vi "api_mqttPublish.vi"(0 "mqtt.lvclass in":refnum<class "mqtt.lvclass">, 5 "topic":string, 7 "value":string, 9 "QoS (At most once)":T3, 11 "error in (no error)":errorcluster, 12 "retain(F)":bool, 13 "duplicate(F)":bool, 14 "messageID":u16) -> (4 "mqtt.lvclass out":refnum<class "mqtt.lvclass">, 6 "success":bool, 15 "error out":errorcluster)   [LabVIEW 2018, in "labview-mqtt.lvlib" / "mqtt.lvclass"]
uses:
  mqtt.lvclass
  mqttTypedef/mqttQOSlevel.ctl
  mqttTypedef/mqttRXdataCluster.ctl
  mqttTypedef/mqttFixedHeaderResponse.ctl
  mqttTypedef/mqttMessageType.ctl
  mqttCmd/mqttCmdPublish/mqttCmdPublish.lvclass
  D:/OneDrive/_WorkingOn/IECube/MQTT LabVIEW/mqtt-LabVIEW-master-yao/src/class/mqtt/mqttCmd/mqttCmd.lvclass
  mqttCmd/mqttCmdPublish/mqttCmdPublish.lvclass/mqttCmdPublish.ctl
  mqttCmd/mqttCmd.lvclass/mqttCmd.ctl
  mqttCmd/mqttCmd.lvclass
  labview-mqtt.lvlib
panel:
  out "notification":T1
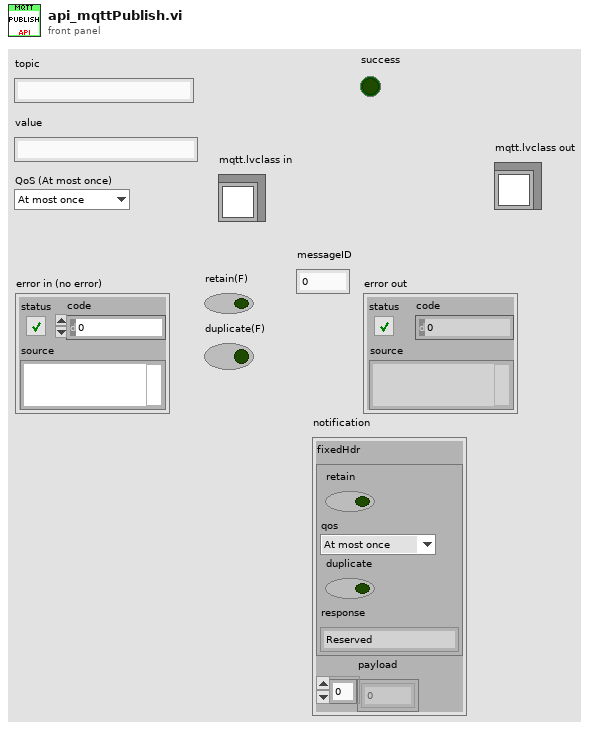
[diagram p1: front panel]
types:
  T1 = typedef "labview-mqtt.lvlib/mqttRXdataCluster.ctl" = cluster{"fixedHdr":T2, "payload":u8[]}
  T2 = typedef "labview-mqtt.lvlib/mqttFixedHeaderResponse.ctl" = cluster{"retain":bool, "qos":T3, "duplicate":bool, "response":T4}
  T3 = typedef "labview-mqtt.lvlib/mqttQOSlevel.ctl" = enum8{"At most once", "At least once", "Exactly once", "Reserved"}
  T4 = typedef "labview-mqtt.lvlib/mqttMessageType.ctl" = enum32{"Reserved", "CONNECT", "CONNACK", "PUBLISH", "PUBACK", "PUBREC", "PUBREL", "PUBCOMP", "SUBSCRIBE", "SUBACK", "UNSUBSCRIBE", "UNSUBACK", "PINGREQ", "PINGRESP", "DISCONNECT", "Reserved2"}
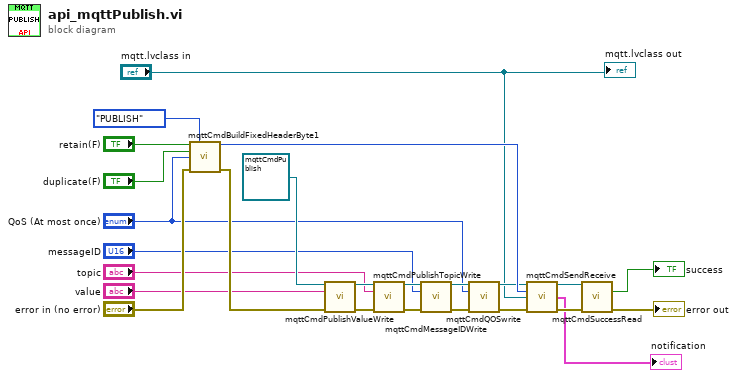
[diagram p0: block diagram]
diagram:
  n1 = call "mqttCmdBuildFixedHeaderByte1.vi"("retain(F)"="retain(F)", "MessageType"=mqttMessageType."PUBLISH", "duplicate(F)"="duplicate(F)", "QoS (At most once)"="QoS (At most once)", "error in (no error)"="error in (no error)") -> ("byte1"=w24:u8, "error out"=w20:errorcluster)  [unwired: 9 in]
  n2 = call "mqttCmdPublishValueWrite.vi"("mqttPublish in"=refnum<class "mqttCmdPublish.lvclass"> refnum ("mqttPublish.lvclass"), "value"="value", "error in (no error)"=w20) -> ("mqttPublish out"=w17:refnum<class "mqttCmdPublish.lvclass">, "error out"=w19:errorcluster)  [unwired: 11 in]
  n3 = call "mqttCmdPublishTopicWrite.vi"("mqttPublish in"=w17, "topic"="topic", "error in (no error)"=w19) -> ("mqttPublish out"=w11:refnum<class "mqttCmdPublish.lvclass">, "error out"=w12:errorcluster)  [unwired: 11 in]
  n4 = call "mqttCmdMessageIDWrite.vi"("mqttBrokerCommand in"=w11, "messageID"="messageID", "error in (no error)"=w12) -> ("mqttBrokerCommand out"=w7:refnum<class "mqttCmdPublish.lvclass">, "error out"=w9:errorcluster)  [unwired: 11 in]
  n5 = call "mqttCmdQOSwrite.vi"("mqttBrokerCommand in"=w7, "QoS"="QoS (At most once)", "error in (no error)"=w9) -> ("mqttBrokerCommand out"=w6:refnum<class "mqttCmdPublish.lvclass">, "error out"=w8:errorcluster)  [unwired: 11 in]
  n6 = call "mqttCmdSendReceive.vi"("mqttConnect in"=w6, "byte1"=w24, "mqtt in"="mqtt.lvclass in", "error in (no error)"=w8) -> ("mqttConnect out"=w4:refnum<class "mqttCmdPublish.lvclass">, "notification"=→"notification":T1, "error out"=w3:errorcluster)  [unwired: 9 in]
  n7 = call "mqttCmdSuccessRead.vi"("mqttBrokerCommand in"=w4, "error in (no error)"=w3) -> ("success"=→"success":bool, "error out"=→"error out":errorcluster)  [unwired: 11 in, 1 out]
  "mqtt.lvclass out" <- "mqtt.lvclass in"
